vi "Get Entire Tree.vi"(0 "Tree Reference In":refnum<vi>, 5 "error in (no error)":errorcluster, 7 "# of Columns":u8) -> (14 "Tree Reference Out":refnum<vi>, 17 "Tree Data":T1[](array[typedef]), 19 "error out":errorcluster)   [LabVIEW 2015, in "QuickVIew.lvlib"]
doc: "Reads all the tags and the following properties for each tag\n[cell strings (For given columns number), Child Only Mode, Item Indent Level, \nLeft Cell String]TLB Prime - Application Template 1.3.0.24\nNorm Kirchner, NI Systems Engineering - NI\nCopyright (c) 2014, NI"
uses:
  QuickVIew.lvlib
  Typedef/TYPEDEF - Tree Item.ctl
panel:
  # "VI LOCALS"
  # "VI OUTPUTS"
  # "VI INPUTS"
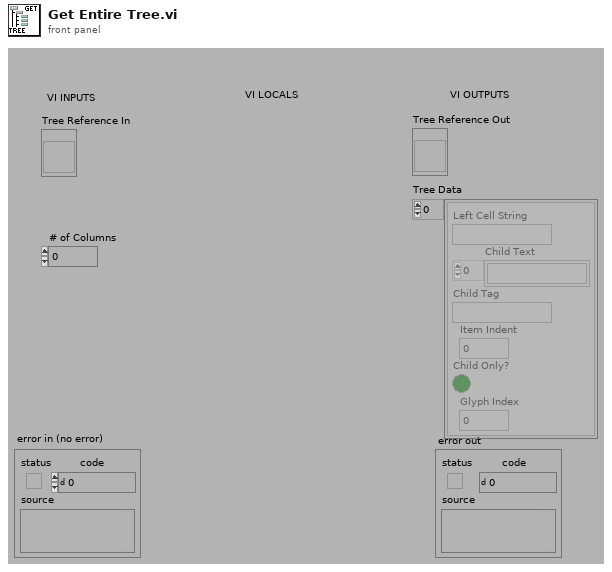
[diagram p1: front panel]
types:
  T1 = typedef "QuickVIew.lvlib/TYPEDEF - Tree Item.ctl" = cluster{"Left Cell String":string, "Child Text":string[], "Child Tag":string, "Item Indent":i32, "Child Only?":bool, "Glyph Index":i32}
  T2 = cluster{"Left Cell String":string, "Child Text":string[], "Child Tag":string, "Item Indent":i32, "Child Only?":bool, "Glyph Index":i32}
  T3 = cluster{"Left Cell String":string, "Child Text":string[], "Child Tag":string, "Item Indent":i32, "Child Only?":bool, "Glyph Index":i32}[]
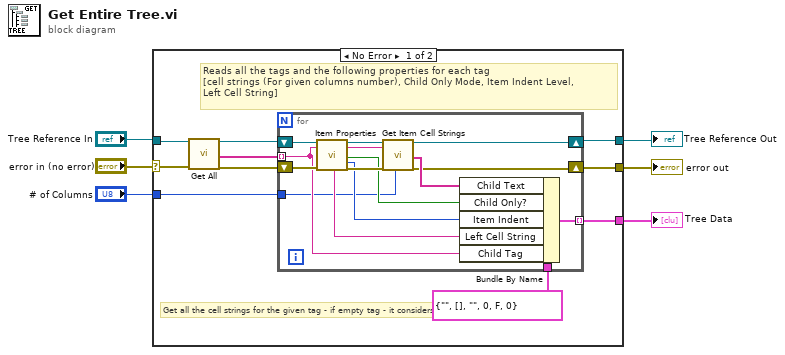
[diagram p0: block diagram]
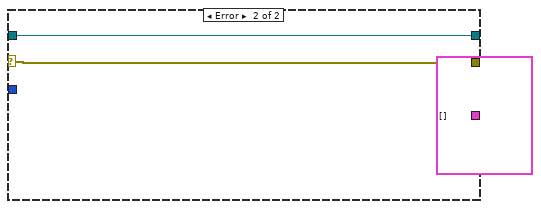
[diagram p2: hidden frame]
diagram:
  # "Get all the cell strings for the given tag - if empty tag - it considers the current tag"
  n1 = case shown="No Error" "error in (no error)" {
    selector: "error in (no error)" -> [w13 w33]
    tunnel: "Tree Reference In" -> [w14 w34]
    tunnel: [w16 w34] -> w5
    tunnel: [w15 w33] -> w4
    tunnel: [w8 T3 []] -> w3
    tunnel: "# of Columns" -> [w7 _]
    frame No Error {
      # "Reads all the tags and the following properties for each tag\n[cell strings (For given columns number), Child Only Mode, Item Indent Level, \nLeft Cell String]"
      n2 = call "Get All.vi"("Tree Reference In"=w14, "error in (no error)"=w13) -> ("Tree Reference Out"=w11:refnum<vi>, "Output Tree Items"=w10:string[], "error out"=w12:errorcluster)  [unwired: 14 in, 1 out]
      n3 = for {
        shift-right: [w18] -> w16
        shift-left: w11 -> [w30]
        shift-right: [w19] -> w15
        shift-left: w12 -> [w31]
        tunnel: w10 -> [w23] mode=indexing
        tunnel: T2 {"Left Cell String"="", "Child Text"=[], "Child Tag"="", "Item Indent"=0, "Child Only?"=FALSE, "Glyph Index"=0} ("Item") -> [w26]
        tunnel: [w20] -> w8 mode=indexing
        tunnel: w7 -> [w17]
        n4 = call "Item Properties.vi"("Tree Reference In"=w30, "Tag (Current)"=w23, "error in (no error)"=w31) -> ("Cell String"=w25:string, "Tree Reference Out"=w27:refnum<vi>, "Duplicate Tag"=w29:string, "Child-Only?"=w21:bool, "Indent Level"=w22:i32, "error out"=w28:errorcluster)  [unwired: 9 in, 2 out]
        n5 = call "Get Item Cell Strings.vi"("Tree Reference In"=w27, "Tag (Current)"=w29, "error in (no error)"=w28, "# of Columns"=w17) -> ("Tree Reference Out"=w18:refnum<vi>, "Cell Strings"=w24:string[], "error out"=w19:errorcluster)  [unwired: 11 in, 2 out]
        n6 = Bundle By Name(cluster=w26, "Child Text"=w24, "Child Only?"=w21, "Item Indent"=w22, "Left Cell String"=w25, "Child Tag"=w23) -> (w20:T2)
      }
    }
    frame Error {
    }
  }
  "error out" <- w4
  "Tree Reference Out" <- w5
  "Tree Data" <- w3
